vi "Decrement Preset Index.vi"(8 "error in (no error)":errorcluster, 11 "MKS MW in":refnum<class "PL MKS MW.lvclass">) -> (0 "error out":errorcluster, 3 "MKS MW out":refnum<class "PL MKS MW.lvclass">)   [LabVIEW 2015, in "PL MKS MW.lvclass"]
doc: "Decrements capacitor position preset index."
uses:
  PL MKS MW.lvclass
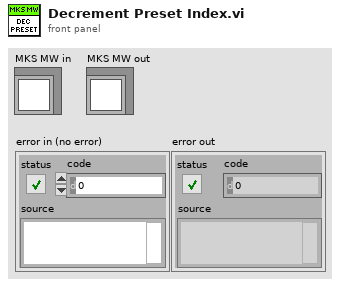
[diagram p1: front panel]
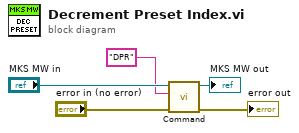
[diagram p0: block diagram]
diagram:
  n1 = call "Command.vi"("error in (no error)"="error in (no error)", "command"="DPR", "MKS MW in"="MKS MW in") -> ("error out"=→"error out":errorcluster, "MKS MW out"=→"MKS MW out":refnum<class "PL MKS MW.lvclass">)  [unwired: 6 in, 1 out]
